vi "JK_flip-flop.vi"(0 "K":bool, 2 "J":bool) -> (7 "Q":bool, 9 "-Q":bool)   [LabVIEW 2019]
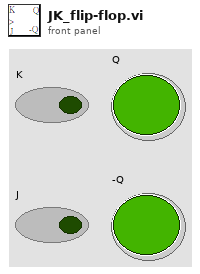
[diagram p1: front panel]
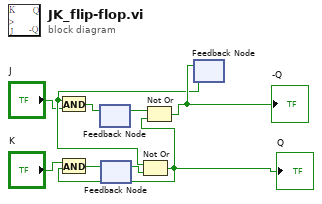
[diagram p0: block diagram]
diagram:
  n1 = feedback #1() -> (w5:bool)  [unwired: 1 in]
  n2 = feedback #2() -> (w6:bool)  [unwired: 1 in]
  n3 = feedback #3() -> (w7:bool)  [unwired: 1 in]
  n4 = And(x=w7, y="J") -> (x .and. y?=w1:bool)
  n5 = feedback-in #1(w1) -> ()
  n6 = Not Or(1:w6, 2:w7) -> (0:w9:bool)
  "Q" <- w9
  n7 = And(x="K", y=w9) -> (x .and. y?=w2:bool)
  n8 = feedback-in #2(w2) -> ()
  n9 = Not Or(1:w9, 2:w5) -> (0:w8:bool)
  "-Q" <- w8
  n10 = feedback-in #3(w8) -> ()
